vi "cube Controller.vi"(8 "error in":errorcluster) -> ()   [LabVIEW 2017]
doc: "This VI executes continuously carrying out the current operation and responding to updates or new operations. It will often contain the timing or control code that is difficult to place directly in TeleOp. This VI generally opens all sensors and motors and isolates the rest of the robot code from knowing how the operations are carried out."
uses:
  <vilib>/Rock Robotics/WPI/Framework/Completion Status.ctl
  cube Setpoints.ctl
  cube Operations.ctl
  <vilib>/Rock Robotics/SystemInterfaces/AI/FPGA_AIChannel.ctl
  Public/Documents/Cross The Road Electronics/Phoenix-LabVIEW/Motor Controller/Controls/CTRE_Phoenix_MotorControl_ControlMode.ctl
  cube Published Globals.vi
  Framework/Robot Global Data.vi
  <vilib>/Rock Robotics/Network Tables/NT Write Boolean.vi
panel:
  out "CubeLastCommandStatus":T1=enum."Incomplete"
  out "WaitTrigger":bool
  in  "Interactive Values":T2
  out "Current\nCmd":string
  in  "Buttons":cluster{"Execute Cmd":bool, "Abort Cmd":bool}
  out "Command Timing":cluster{"Start Time (ms)":u32, "Iterations":i32}
  out "Status":T1
  # "Tip: It may be helpful to observe inputs and sensor values.\nYou may also want to display tuning or debugging controls."
  # "Interactive Command: You may fill in the settings for a command\nand schedule it with the Execute button. You can observe and abort\nany command while fine tuning the code for the controller."
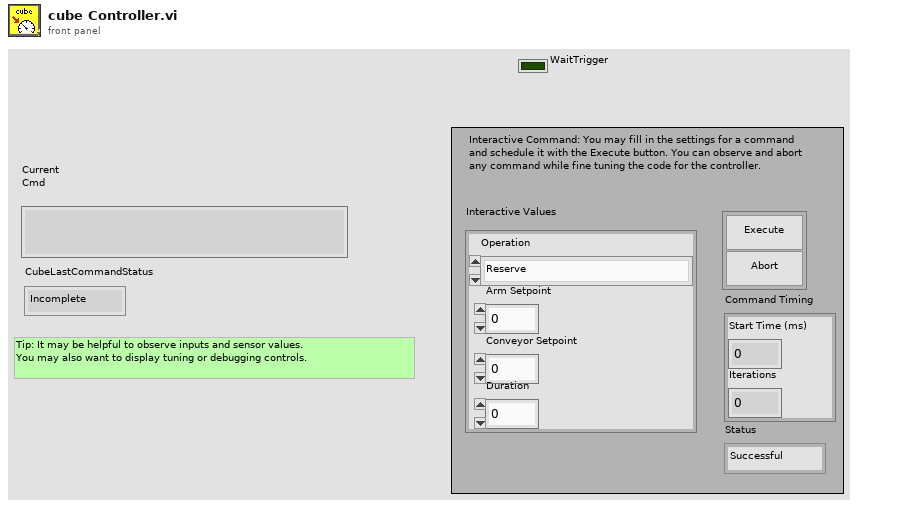
[diagram p1: front panel]
types:
  T1 = typedef "Completion Status.ctl" = enum16{"Successful", "Aborted", "Incomplete"}
  T2 = typedef "cube Setpoints.ctl" = cluster{"Operation":T3, "Arm Setpoint":dbl, "Duration":dbl, "Conveyor Setpoint":dbl}
  T3 = typedef "cube Operations.ctl" = enum16{"Reserve", "Read Current", "Immediate", "Chew", "Puke", "Swallow", "Poop", "SpitFast", "SpitSlow"}
  T4 = typedef "FPGA_AIChannel.ctl" = enum8{"AI 0", "AI 1", "AI 2", "AI 3", "AI MXP 0", "AI MXP 1", "AI MXP 2", "AI MXP 3", "Invalid"}
  T5 = typedef "WPI_AnalogChannelDevRef.ctl" = cluster{"DevStatus":errorcluster, "Analog Channel":T4}
  T6 = typedef "WPI_MotorControlDeviceRef.ctl" = cluster{"DeviceStatus":errorcluster, "Type":T7, "PWM":cluster{"PWM Channel":T8, "DeadBand":T9}, "CAN":cluster{"Device Number":u8, "SetOutput VI Ref":variant, "GetOutput VI Ref":variant, "Enable VI Ref":variant, "Disable VI Ref":variant, "Data":variant}, "Invert":bool, "DIO PWM":cluster{"PWM \"Enable\" Channel":T8, "DIOChannel":T10, "PWM Rate":dbl}}
  T7 = typedef "WPI_MotorControlType.ctl" = enum16{"PWM", "CAN", "DIO PWM"}
  T8 = typedef "FPGA_DIOPWMChannel.ctl" = enum8{"PWM 0", "PWM 1", "PWM 2", "PWM 3", "PWM 4", "PWM 5", "PWM 6", "PWM 7", "PWM 8", "PWM 9", "PWM MXP 0", "PWM MXP 1", "PWM MXP 2", "PWM MXP 3", "PWM MXP 4", "PWM MXP 5", "PWM MXP 6", "PWM MXP 7", "PWM MXP 8", "PWM MXP 9", "Invalid"}
  T9 = typedef "WPI_PWMDeadband.ctl" = cluster{"Name":string, "maxPositivePwm":i32, "minPositivePwm":i32, "centerPwm":i32, "maxNegativePwm":i32, "minNegativePwm":i32, "angularRange":u16}
  T10 = typedef "FPGA_DIOChannel.ctl" = enum8{"DIO 0", "DIO 1", "DIO 2", "DIO 3", "DIO 4", "DIO 5", "DIO 6", "DIO 7", "DIO 8", "DIO 9", "DIO MXP 0", "DIO MXP 1", "DIO MXP 2", "DIO MXP 3", "DIO MXP 4", "DIO MXP 5", "DIO MXP 6", "DIO MXP 7", "DIO MXP 8", "DIO MXP 9", "DIO MXP 10", "DIO MXP 11", "DIO MXP 12", "DIO MXP 13", "DIO MXP 14", "DIO MXP 15", "SPI Port CS1", "SPI Port CS2", "SPI Port CS3", "SPI Port MISO", "SPI Port MOSI", "Invalid"}
  T11 = typedef "FPGA_AnalogTriggerDevRef.ctl" = cluster{"DevStatus":errorcluster, "AnalogTriggerIndex":T12}
  T12 = typedef "FPGA_AnalogTriggerIndex.ctl" = enum8{"Trig 0", "Trig 1", "Trig 2", "Trig 3", "Trig 4", "Trig 5", "Trig 6", "Trig 7", "Invalid"}
  T13 = typedef "Command Status Info.ctl" = cluster{"Name":string, "Status":T1, "notifier out":T14}
  T14 = typedef "Completion Notifier.ctl" = refnum<notifier>
  T15 = cluster{"Current Command":T2, "Command Timing":cluster{"Start Time (ms)":u32, "Iterations":i32}, "Command Arguments":cluster{"Command Info":T13, "Description":string, "Default Command":T2, "queue out":refnum<queue>, "Subsystem Name":string}}
  T16 = typedef "CTRE_Phoenix_MotorControl_ControlMode.ctl" = u16
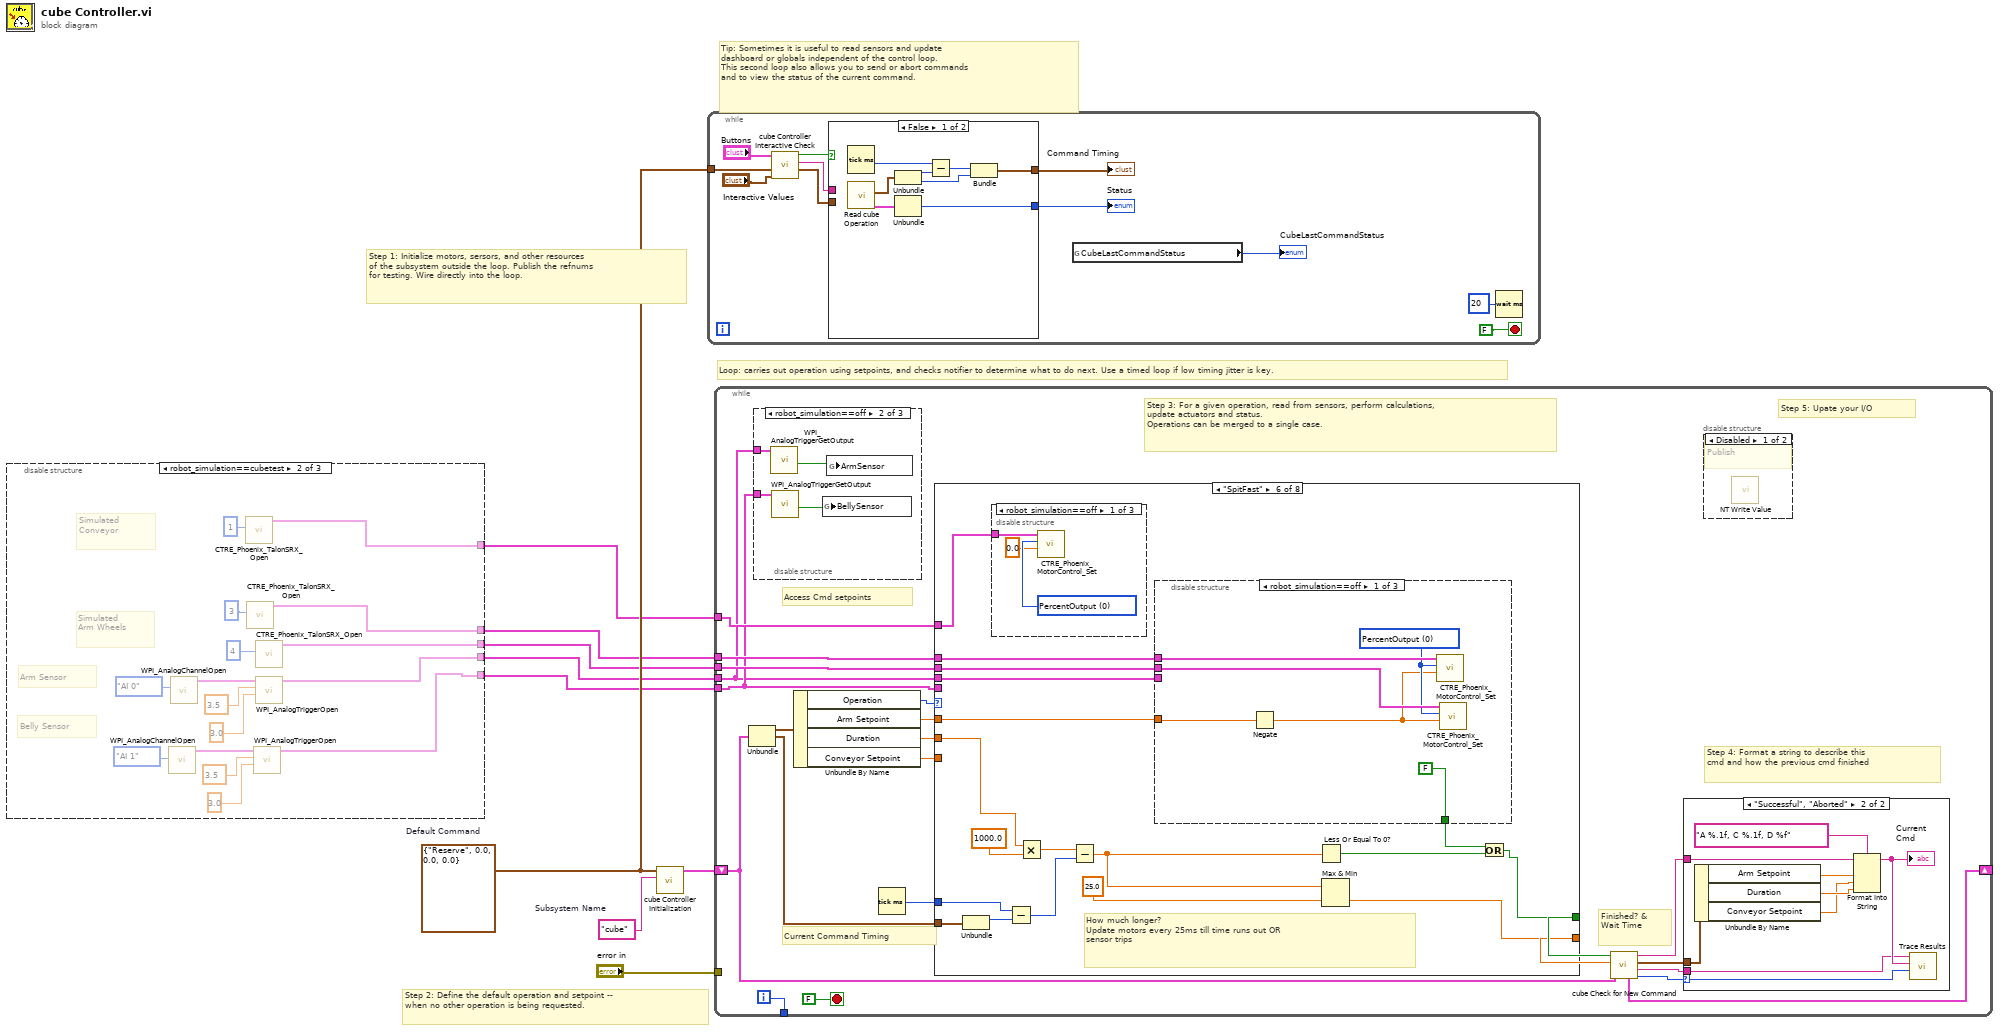
[diagram p0: block diagram]
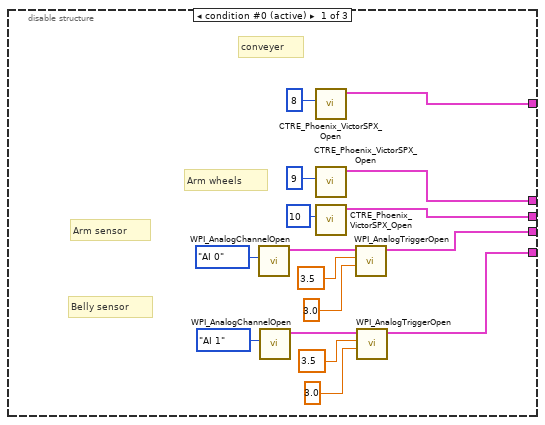
[diagram p2: hidden frame]
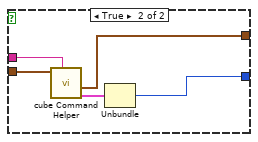
[diagram p4: hidden frame]
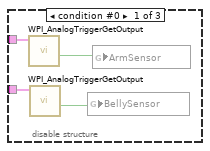
[diagram p5: hidden frame]
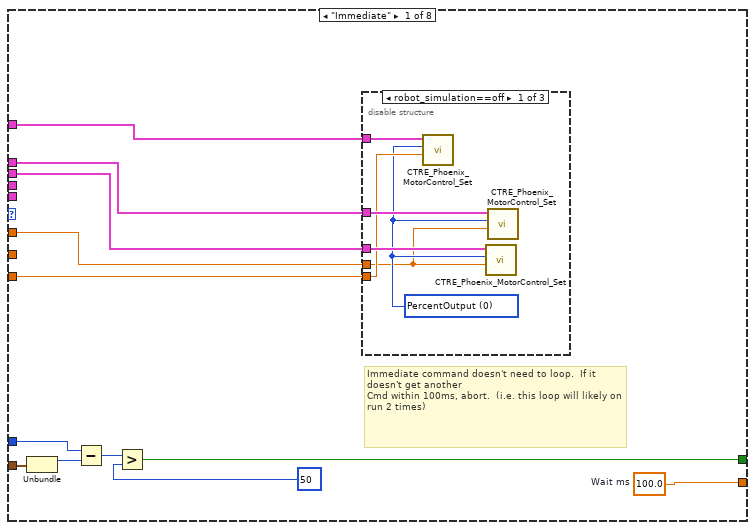
[diagram p9: hidden frame]
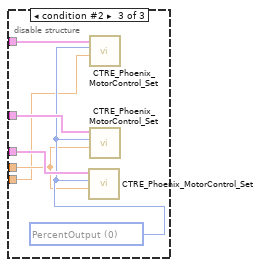
[diagram p11: hidden frame]
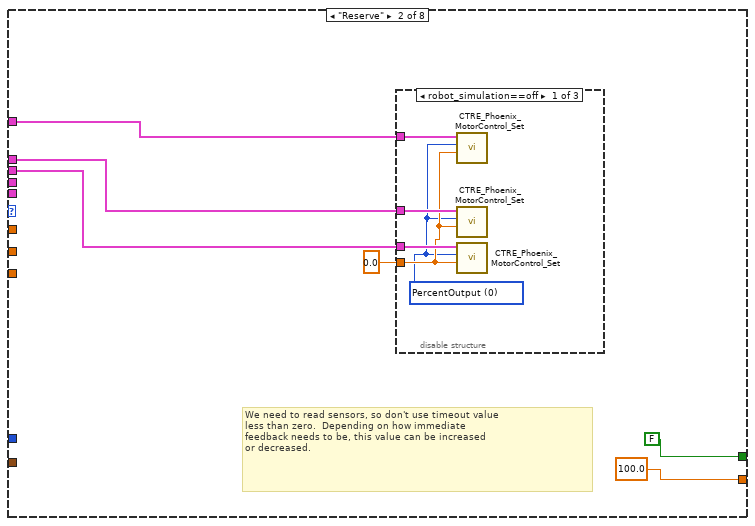
[diagram p12: hidden frame]
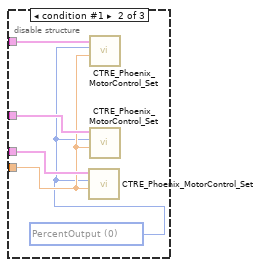
[diagram p13: hidden frame]
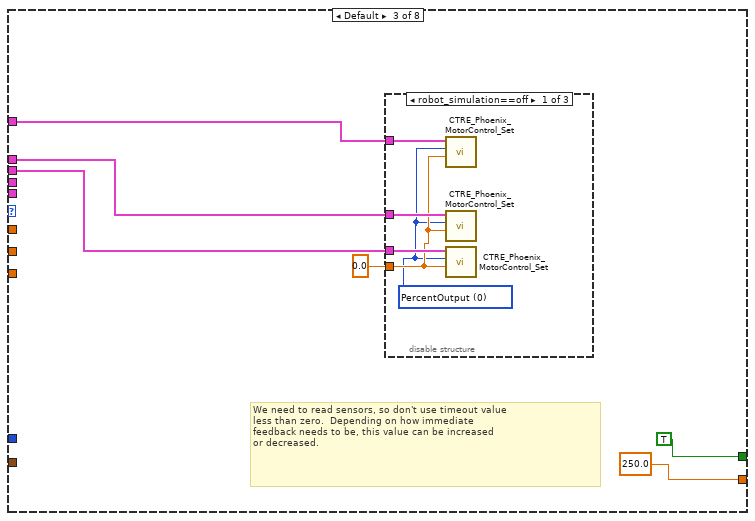
[diagram p15: hidden frame]
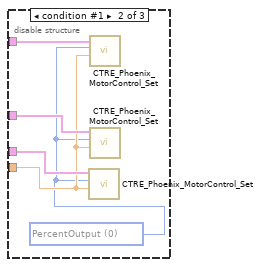
[diagram p16: hidden frame]
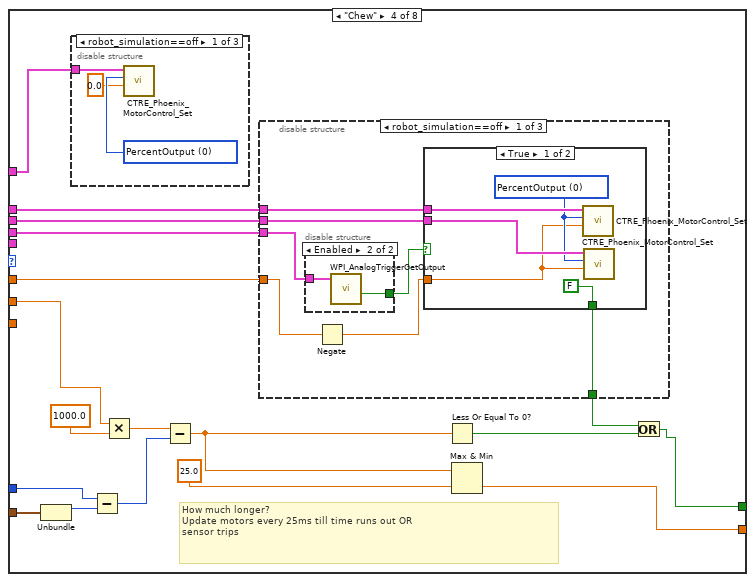
[diagram p18: hidden frame]
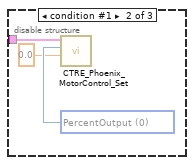
[diagram p19: hidden frame]
diagram:
  w6 = T2 {"Operation"=enum."Reserve", "Arm Setpoint"=0.0, "Duration"=0.0, "Conveyor Setpoint"=0.0}  # Default Command
  w7 = "cube"  # Subsystem Name
  # "Tip: Sometimes it is useful to read sensors and update\ndashboard or globals independent of the control loop.\nThis second loop also allows you to send or abort commands\nand to view the status of the current command."
  # "Step 2: Define the default operation and setpoint --\nwhen no other operation is being requested."
  # "Step 1: Initialize motors, sersors, and other resources\nof the subsystem outside the loop. Publish the refnums\nfor testing. Wire directly into the loop."
  # "Loop: carries out operation using setpoints, and checks notifier to determine what to do next. Use a timed loop if low timing jitter is key."
  n1 = disable-structure shown="robot_simulation==cubetest" {
    disable-tunnel: [w22 w38 _] -> w5
    disable-tunnel: [w21 w37 _] -> w4
    disable-tunnel: [w10 w36 _] -> w1
    disable-tunnel: [w16 w31 _] -> w3
    disable-tunnel: [w11 w26 _] -> w2
    frame condition #0 (active) {
      # "Belly sensor"
      # "Arm sensor"
      # "Arm wheels"
      # "conveyer"
      n2 = call <vilib>:"WPI_AnalogChannelOpen.vi"("Analog Channel"=FPGA_AIChannel."AI 0") -> ("AIDeviceRef"=w19:T5)  [unwired: 9 in, 1 out]
      n3 = call <vilib>:"WPI_AnalogChannelOpen.vi"("Analog Channel"=FPGA_AIChannel."AI 1") -> ("AIDeviceRef"=w14:T5)  [unwired: 9 in, 1 out]
      n4 = call "CTRE_Phoenix_VictorSPX_Open.vi"("Device Number"=u8 8) -> ("CAN Talon SRX Ref"=w10:T6)  [unwired: 9 in, 1 out]
      n5 = call "CTRE_Phoenix_VictorSPX_Open.vi"("Device Number"=u8 9) -> ("CAN Talon SRX Ref"=w22:T6)  [unwired: 9 in, 1 out]
      n6 = call "CTRE_Phoenix_VictorSPX_Open.vi"("Device Number"=u8 10) -> ("CAN Talon SRX Ref"=w21:T6)  [unwired: 9 in, 1 out]
      n7 = call <vilib>:"WPI_AnalogTriggerOpen.vi"("LowerLimit (v)"=3.0, "UpperLimit (v)"=3.5, "AnalogTriggerSource"=w19) -> ("AnalogTriggerDevRef"=w16:T11)  [unwired: 7 in, 1 out]
      n8 = call <vilib>:"WPI_AnalogTriggerOpen.vi"("LowerLimit (v)"=3.0, "UpperLimit (v)"=3.5, "AnalogTriggerSource"=w14) -> ("AnalogTriggerDevRef"=w11:T11)  [unwired: 7 in, 1 out]
    }
    frame condition #1 {
      # "Belly Sensor"
      # "Arm Sensor"
      # "Simulated\nConveyor"
      # "Simulated\nArm Wheels"
      n9 = call <vilib>:"WPI_AnalogChannelOpen.vi"("Analog Channel"=FPGA_AIChannel."AI 1") -> ("AIDeviceRef"=w29:T5)  [unwired: 9 in, 1 out]
      n10 = call <vilib>:"WPI_AnalogChannelOpen.vi"("Analog Channel"=FPGA_AIChannel."AI 0") -> ("AIDeviceRef"=w34:T5)  [unwired: 9 in, 1 out]
      n11 = call "CTRE_Phoenix_TalonSRX_Open.vi"("Device Number"=u8 1) -> ("CAN Talon SRX Ref"=w36:T6)  [unwired: 9 in, 1 out]
      n12 = call "CTRE_Phoenix_TalonSRX_Open.vi"("Device Number"=u8 3) -> ("CAN Talon SRX Ref"=w38:T6)  [unwired: 9 in, 1 out]
      n13 = call <vilib>:"WPI_AnalogTriggerOpen.vi"("LowerLimit (v)"=3.0, "UpperLimit (v)"=3.5, "AnalogTriggerSource"=w29) -> ("AnalogTriggerDevRef"=w26:T11)  [unwired: 7 in, 1 out]
      n14 = call "CTRE_Phoenix_TalonSRX_Open.vi"("Device Number"=u8 4) -> ("CAN Talon SRX Ref"=w37:T6)  [unwired: 9 in, 1 out]
      n15 = call <vilib>:"WPI_AnalogTriggerOpen.vi"("LowerLimit (v)"=3.0, "UpperLimit (v)"=3.5, "AnalogTriggerSource"=w34) -> ("AnalogTriggerDevRef"=w31:T11)  [unwired: 7 in, 1 out]
    }
    frame condition #2 {
    }
  }
  n16 = call "cube Controller Initialization.vi"("Subsystem Name"=w7, "Default Command"=w6) -> ("Current Command"=w8:T15)  [unwired: 9 in]
  n17 = while {
    tunnel: w6 -> [w49]
    stop <- FALSE stop-if-true
    n18 = call "cube Controller Interactive Check.vi"("Interactive Command in"="Interactive Values", "Default Command"=w49, "Buttons"="Buttons") -> ("Interactive Command out"=w46:T2, "Trace String"=w47:string, "Schedule"=w48:bool)  [unwired: 6 in]
    n19 = case shown="False" w48 {
      tunnel: [w60 w65] -> w45
      tunnel: w46 -> [_ w63]
      tunnel: [w56 w61] -> w44
      tunnel: w47 -> [_ w64]
      frame False {
        n20 = Tick Count (ms)() -> (millisecond timer value=w55:u32)
        n21 = call "Read cube Operation.vi"() -> ("Command Info"=w54:T13, "Command Timing"=w53:cluster{"Start Time (ms)":u32, "Iterations":i32})  [unwired: 9 in, 1 out]
        n22 = Unbundle(w53) -> ("Start Time (ms)"=w59:u32, "Iterations"=w57:i32)
        n23 = Unbundle(w54) -> ("Status"=w60:T1)  [unwired: 2 out]
        n24 = Subtract(x=w55, y=w59) -> (x-y=w58:u32)
        n25 = Bundle(w58, "Iterations"=w57) -> (w56:cluster{u32, "Iterations":i32})  [unwired: 1 in]
      }
      frame True {
        n26 = call "cube Command Helper.vi"("Description"=w64, "SubSystem Data"=w63) -> ("Command Info Out"=w62:T13, "Command Timing"=w61:cluster{"Start Time (ms)":u32, "Iterations":i32})  [unwired: 7 in, 1 out]
        n27 = Unbundle(w62) -> ("Status"=w65:T1)  [unwired: 2 out]
      }
    }
    "Status" <- w45
    "Command Timing" <- w44
    n28 = global read "cube Published Globals.vi" "CubeLastCommandStatus"() -> (→"CubeLastCommandStatus":T1)
    n29 = Wait (ms)(milliseconds to wait=u32 20) -> ()  [unwired: 1 out]
  }
  n30 = while {
    shift-right: [w83] -> _
    shift-left: w8 -> [w76]
    tunnel: [w86] -> _
    tunnel: "error in" -> [_]
    tunnel: w5 -> [w75]
    tunnel: w4 -> [w74]
    tunnel: w1 -> [w73]
    tunnel: w3 -> [w66]
    tunnel: w2 -> [w67]
    i -> [w86]
    stop <- FALSE stop-if-true
    # "Step 5: Upate your I/O"
    # "Step 4: Format a string to describe this\ncmd and how the previous cmd finished"
    # "Current Command Timing"
    # "Access Cmd setpoints"
    # "Finished? &\nWait Time"
    # "Step 3: For a given operation, read from sensors, perform calculations,\nupdate actuators and status.\nOperations can be merged to a single case."
    n31 = Unbundle(w76) -> ("Current Command"=w72:T2, "Command Timing"=w84:cluster{"Start Time (ms)":u32, "Iterations":i32})  [unwired: 1 out]
    n32 = disable-structure shown="robot_simulation==off" {
      disable-tunnel: w67 -> [w88 w93 _]
      disable-tunnel: w66 -> [w89 w92 _]
      frame condition #0 {
        n33 = call <vilib>:"WPI_AnalogTriggerGetOutput.vi"("AnalogTriggerDevRef"=w89) -> ("Trigger State"=w91:bool)  [unwired: 7 in, 3 out]
        n34 = call <vilib>:"WPI_AnalogTriggerGetOutput.vi"("AnalogTriggerDevRef"=w88) -> ("Trigger State"=w90:bool)  [unwired: 7 in, 3 out]
        n35 = global write "Robot Global Data.vi" "BellySensor"(w90) -> ()
        n36 = global write "Robot Global Data.vi" "ArmSensor"(w91) -> ()
      }
      frame condition #1 (active) {
        n37 = call <vilib>:"WPI_AnalogTriggerGetOutput.vi"("AnalogTriggerDevRef"=w92) -> ("Trigger State"=w95:bool)  [unwired: 7 in, 3 out]
        n38 = call <vilib>:"WPI_AnalogTriggerGetOutput.vi"("AnalogTriggerDevRef"=w93) -> ("Trigger State"=w94:bool)  [unwired: 7 in, 3 out]
        n39 = global write "Robot Global Data.vi" "BellySensor"(w94) -> ()
        n40 = global write "Robot Global Data.vi" "ArmSensor"(w95) -> ()
      }
      frame condition #2 {
      }
    }
    n41 = Unbundle By Name(w72) -> ("Operation"=w71:T3, "Arm Setpoint"=w70:dbl, "Duration"=w69:dbl, "Conveyor Setpoint"=w68:dbl)
    n42 = Tick Count (ms)() -> (millisecond timer value=w85:u32)
    n43 = case shown="\"SpitFast\"" w71 {
      tunnel: [w116 100.0 250.0 ("Infinite") w170 w231 w267 w304 w372] -> w81
      tunnel: [w110 FALSE ("ignore previous (F)") TRUE ("ignore previous (F)") w165 w227 w262 w300 w368] -> w82
      tunnel: w84 -> [w112 _ _ w172 w233 w269 w306 w374]
      tunnel: w85 -> [w111 _ _ w171 w232 w268 w305 w373]
      tunnel: w75 -> [w108 w131 w147 w169 w230 w266 w303 w371]
      tunnel: w74 -> [w107 w130 w146 w168 w229 w265 w302 w370]
      tunnel: w73 -> [w109 w132 w148 w161 w222 w258 w295 w364]
      tunnel: w70 -> [w106 _ _ w162 w224 w259 w297 w365]
      tunnel: w69 -> [_ _ _ w167 w228 w264 w301 w369]
      tunnel: w68 -> [w105 _ _ _ w221 _ w294 w363]
      tunnel: w66 -> [_ _ _ w166 _ w263 _ w358]
      tunnel: w67 -> [_ _ _ _ w223 _ w296 w362]
      frame "Immediate" {
        w116 = 100.0  # Wait ms
        # "Immediate command doesn't need to loop.  If it doesn't get another\nCmd within 100ms, abort.  (i.e. this loop will likely on run 2 times)"
        n44 = Unbundle(w112) -> ("Start Time (ms)"=w115:u32)  [unwired: 1 out]
        n45 = Subtract(x=w111, y=w115) -> (x-y=w114:u32)
        n46 = Greater?(x=w114, y=u8 50 ("Left Motor")) -> (0:w110:bool)
        n47 = disable-structure shown="robot_simulation==off" {
          disable-tunnel: w109 -> [w122 _ w128]
          disable-tunnel: w108 -> [w121 _ w127]
          disable-tunnel: w107 -> [w120 _ w126]
          disable-tunnel: w106 -> [w117 _ w124]
          disable-tunnel: w105 -> [w119 _ w123]
          frame condition #0 (active) {
            w118 = T16 0 items=["PercentOutput"=0, "Position"=1, "Velocity"=2, "Current"=3, "Follower"=5, "MotionProfile"=6, "MotionMagic"=7, "MotionMagicArc"=8, "MotionProfileArc"=10, "Disabled"=15] ("Control Mode")
            n48 = call "CTRE_Phoenix_MotorControl_Set.vi"("Output"=w119, "Control Mode"=w118, "PhoenixMotorControlDevRef"=w122) -> ()  [unwired: 7 in, 2 out]
            n49 = call "CTRE_Phoenix_MotorControl_Set.vi"("Output"=w117, "Control Mode"=w118, "PhoenixMotorControlDevRef"=w120) -> ()  [unwired: 7 in, 2 out]
            n50 = call "CTRE_Phoenix_MotorControl_Set.vi"("Output"=w117, "Control Mode"=w118, "PhoenixMotorControlDevRef"=w121) -> ()  [unwired: 7 in, 2 out]
          }
          frame condition #1 {
          }
          frame condition #2 {
            w125 = T16 0 items=["PercentOutput"=0, "Position"=1, "Velocity"=2, "Current"=3, "Follower"=5, "MotionProfile"=6, "MotionMagic"=7, "MotionMagicArc"=8, "MotionProfileArc"=10, "Disabled"=15] ("Control Mode")
            n51 = call "CTRE_Phoenix_MotorControl_Set.vi"("Output"=w124, "Control Mode"=w125, "PhoenixMotorControlDevRef"=w126) -> ()  [unwired: 7 in, 2 out]
            n52 = call "CTRE_Phoenix_MotorControl_Set.vi"("Output"=w123, "Control Mode"=w125, "PhoenixMotorControlDevRef"=w128) -> ()  [unwired: 7 in, 2 out]
            n53 = call "CTRE_Phoenix_MotorControl_Set.vi"("Output"=w124, "Control Mode"=w125, "PhoenixMotorControlDevRef"=w127) -> ()  [unwired: 7 in, 2 out]
          }
        }
      }
      frame "Reserve" {
        # "We need to read sensors, so don't use timeout value\nless than zero.  Depending on how immediate \nfeedback needs to be, this value can be increased\nor decreased."
        n54 = disable-structure shown="robot_simulation==off" {
          disable-tunnel: w132 -> [w139 w144 _]
          disable-tunnel: w131 -> [w138 w143 _]
          disable-tunnel: w130 -> [w137 w142 _]
          disable-tunnel: 0.0 ("Setpoint") -> [w136 w141 _]
          frame condition #0 (active) {
            w135 = T16 0 items=["PercentOutput"=0, "Position"=1, "Velocity"=2, "Current"=3, "Follower"=5, "MotionProfile"=6, "MotionMagic"=7, "MotionMagicArc"=8, "MotionProfileArc"=10, "Disabled"=15] ("Control Mode")
            n55 = call "CTRE_Phoenix_MotorControl_Set.vi"("Output"=w136, "Control Mode"=w135, "PhoenixMotorControlDevRef"=w139) -> ()  [unwired: 7 in, 2 out]
            n56 = call "CTRE_Phoenix_MotorControl_Set.vi"("Output"=w136, "Control Mode"=w135, "PhoenixMotorControlDevRef"=w138) -> ()  [unwired: 7 in, 2 out]
            n57 = call "CTRE_Phoenix_MotorControl_Set.vi"("Output"=w136, "Control Mode"=w135, "PhoenixMotorControlDevRef"=w137) -> ()  [unwired: 7 in, 2 out]
          }
          frame condition #1 {
            w140 = T16 0 items=["PercentOutput"=0, "Position"=1, "Velocity"=2, "Current"=3, "Follower"=5, "MotionProfile"=6, "MotionMagic"=7, "MotionMagicArc"=8, "MotionProfileArc"=10, "Disabled"=15] ("Control Mode")
            n58 = call "CTRE_Phoenix_MotorControl_Set.vi"("Output"=w141, "Control Mode"=w140, "PhoenixMotorControlDevRef"=w142) -> ()  [unwired: 7 in, 2 out]
            n59 = call "CTRE_Phoenix_MotorControl_Set.vi"("Output"=w141, "Control Mode"=w140, "PhoenixMotorControlDevRef"=w144) -> ()  [unwired: 7 in, 2 out]
            n60 = call "CTRE_Phoenix_MotorControl_Set.vi"("Output"=w141, "Control Mode"=w140, "PhoenixMotorControlDevRef"=w143) -> ()  [unwired: 7 in, 2 out]
          }
          frame condition #2 {
          }
        }
      }
      frame Default {
        # "We need to read sensors, so don't use timeout value\nless than zero.  Depending on how immediate \nfeedback needs to be, this value can be increased\nor decreased."
        n61 = disable-structure shown="robot_simulation==off" {
          disable-tunnel: w148 -> [w155 w160 _]
          disable-tunnel: w147 -> [w154 w159 _]
          disable-tunnel: w146 -> [w153 w158 _]
          disable-tunnel: 0.0 ("Setpoint") -> [w152 w157 _]
          frame condition #0 (active) {
            w151 = T16 0 items=["PercentOutput"=0, "Position"=1, "Velocity"=2, "Current"=3, "Follower"=5, "MotionProfile"=6, "MotionMagic"=7, "MotionMagicArc"=8, "MotionProfileArc"=10, "Disabled"=15] ("Control Mode")
            n62 = call "CTRE_Phoenix_MotorControl_Set.vi"("Output"=w152, "Control Mode"=w151, "PhoenixMotorControlDevRef"=w155) -> ()  [unwired: 7 in, 2 out]
            n63 = call "CTRE_Phoenix_MotorControl_Set.vi"("Output"=w152, "Control Mode"=w151, "PhoenixMotorControlDevRef"=w154) -> ()  [unwired: 7 in, 2 out]
            n64 = call "CTRE_Phoenix_MotorControl_Set.vi"("Output"=w152, "Control Mode"=w151, "PhoenixMotorControlDevRef"=w153) -> ()  [unwired: 7 in, 2 out]
          }
          frame condition #1 {
            w156 = T16 0 items=["PercentOutput"=0, "Position"=1, "Velocity"=2, "Current"=3, "Follower"=5, "MotionProfile"=6, "MotionMagic"=7, "MotionMagicArc"=8, "MotionProfileArc"=10, "Disabled"=15] ("Control Mode")
            n65 = call "CTRE_Phoenix_MotorControl_Set.vi"("Output"=w157, "Control Mode"=w156, "PhoenixMotorControlDevRef"=w158) -> ()  [unwired: 7 in, 2 out]
            n66 = call "CTRE_Phoenix_MotorControl_Set.vi"("Output"=w157, "Control Mode"=w156, "PhoenixMotorControlDevRef"=w160) -> ()  [unwired: 7 in, 2 out]
            n67 = call "CTRE_Phoenix_MotorControl_Set.vi"("Output"=w157, "Control Mode"=w156, "PhoenixMotorControlDevRef"=w159) -> ()  [unwired: 7 in, 2 out]
          }
          frame condition #2 {
          }
        }
      }
      frame "Chew" {
        # "How much longer?\nUpdate motors every 25ms till time runs out OR\nsensor trips"
        n68 = Unbundle(w172) -> ("Start Time (ms)"=w175:u32)  [unwired: 1 out]
        n69 = disable-structure shown="robot_simulation==off" {
          disable-tunnel: w161 -> [w180 w183 _]
          frame condition #0 (active) {
            w181 = T16 0 items=["PercentOutput"=0, "Position"=1, "Velocity"=2, "Current"=3, "Follower"=5, "MotionProfile"=6, "MotionMagic"=7, "MotionMagicArc"=8, "MotionProfileArc"=10, "Disabled"=15] ("Control Mode")
            n70 = call "CTRE_Phoenix_MotorControl_Set.vi"("Output"=0.0, "Control Mode"=w181, "PhoenixMotorControlDevRef"=w180) -> ()  [unwired: 7 in, 2 out]
          }
          frame condition #1 {
            w184 = T16 0 items=["PercentOutput"=0, "Position"=1, "Velocity"=2, "Current"=3, "Follower"=5, "MotionProfile"=6, "MotionMagic"=7, "MotionMagicArc"=8, "MotionProfileArc"=10, "Disabled"=15] ("Control Mode")
            n71 = call "CTRE_Phoenix_MotorControl_Set.vi"("Output"=0.0, "Control Mode"=w184, "PhoenixMotorControlDevRef"=w183) -> ()  [unwired: 7 in, 2 out]
          }
          frame condition #2 {
          }
        }
        n72 = Subtract(x=w171, y=w175) -> (x-y=w178:u32)
        n73 = Multiply(x=w167, y=1000.0) -> (x*y=w177:dbl)
        n74 = Subtract(x=w177, y=w178) -> (x-y=w174:dbl)
        n75 = disable-structure shown="robot_simulation==off" {
          disable-tunnel: w169 -> [w191 w210 _]
          disable-tunnel: w168 -> [w190 w209 _]
          disable-tunnel: w162 -> [w185 w208 _]
          disable-tunnel: w166 -> [w189 w207 _]
          disable-tunnel: [w187 w205 _] -> w163
          frame condition #0 (active) {
            n76 = disable-structure shown="Enabled" {
              disable-tunnel: w189 -> [_ w194]
              disable-tunnel: [TRUE ("Trigger State") w193] -> w188
              frame Disabled {
              }
              frame Enabled {
                n77 = call <vilib>:"WPI_AnalogTriggerGetOutput.vi"("AnalogTriggerDevRef"=w194) -> ("Trigger State"=w193:bool)  [unwired: 7 in, 3 out]
              }
            }
            n78 = Negate(x=w185) -> (-x=w186:dbl)
            n79 = case shown="True" w188 {
              tunnel: w191 -> [w199 w204]
              tunnel: w190 -> [w198 w203]
              tunnel: w186 -> [w195 _]
              tunnel: [FALSE TRUE] -> w187
              frame True {
                w197 = T16 0 items=["PercentOutput"=0, "Position"=1, "Velocity"=2, "Current"=3, "Follower"=5, "MotionProfile"=6, "MotionMagic"=7, "MotionMagicArc"=8, "MotionProfileArc"=10, "Disabled"=15] ("Control Mode")
                n80 = call "CTRE_Phoenix_MotorControl_Set.vi"("Output"=w195, "Control Mode"=w197, "PhoenixMotorControlDevRef"=w199) -> ()  [unwired: 7 in, 2 out]
                n81 = call "CTRE_Phoenix_MotorControl_Set.vi"("Output"=w195, "Control Mode"=w197, "PhoenixMotorControlDevRef"=w198) -> ()  [unwired: 7 in, 2 out]
              }
              frame False {
                w201 = 0.0 ("Output")
                w202 = T16 0 items=["PercentOutput"=0, "Position"=1, "Velocity"=2, "Current"=3, "Follower"=5, "MotionProfile"=6, "MotionMagic"=7, "MotionMagicArc"=8, "MotionProfileArc"=10, "Disabled"=15] ("Control Mode")
                n82 = call "CTRE_Phoenix_MotorControl_Set.vi"("Output"=w201, "Control Mode"=w202, "PhoenixMotorControlDevRef"=w204) -> ()  [unwired: 7 in, 2 out]
                n83 = call "CTRE_Phoenix_MotorControl_Set.vi"("Output"=w201, "Control Mode"=w202, "PhoenixMotorControlDevRef"=w203) -> ()  [unwired: 7 in, 2 out]
              }
            }
          }
          frame condition #1 {
            n84 = call <vilib>:"WPI_AnalogTriggerGetOutput.vi"("AnalogTriggerDevRef"=w207) -> ("Trigger State"=w206:bool)  [unwired: 7 in, 3 out]
            n85 = case shown="True" w206 {
              tunnel: w210 -> [w214 w220]
              tunnel: w209 -> [w213 w219]
              tunnel: w208 -> [w211 _]
              tunnel: [FALSE TRUE] -> w205
              frame True {
                w212 = T16 0 items=["PercentOutput"=0, "Position"=1, "Velocity"=2, "Current"=3, "Follower"=5, "MotionProfile"=6, "MotionMagic"=7, "MotionMagicArc"=8, "MotionProfileArc"=10, "Disabled"=15] ("Control Mode")
                n86 = call "CTRE_Phoenix_MotorControl_Set.vi"("Output"=w211, "Control Mode"=w212, "PhoenixMotorControlDevRef"=w214) -> ()  [unwired: 7 in, 2 out]
                n87 = call "CTRE_Phoenix_MotorControl_Set.vi"("Output"=w211, "Control Mode"=w212, "PhoenixMotorControlDevRef"=w213) -> ()  [unwired: 7 in, 2 out]
              }
              frame False {
                w218 = T16 0 items=["PercentOutput"=0, "Position"=1, "Velocity"=2, "Current"=3, "Follower"=5, "MotionProfile"=6, "MotionMagic"=7, "MotionMagicArc"=8, "MotionProfileArc"=10, "Disabled"=15] ("Control Mode")
                w217 = 0.0 ("Output")
                n88 = call "CTRE_Phoenix_MotorControl_Set.vi"("Output"=w217, "Control Mode"=w218, "PhoenixMotorControlDevRef"=w220) -> ()  [unwired: 7 in, 2 out]
                n89 = call "CTRE_Phoenix_MotorControl_Set.vi"("Output"=w217, "Control Mode"=w218, "PhoenixMotorControlDevRef"=w219) -> ()  [unwired: 7 in, 2 out]
              }
            }
          }
          frame condition #2 {
          }
        }
        n90 = Less Or Equal To 0?(x=w174) -> (x <= 0?=w164:bool)
        n91 = Max & Min(x=w174, y=25.0) -> (min(x,y)=w170:dbl)  [unwired: 1 out]
        n92 = Or(x=w163, y=w164) -> (x .or. y?=w165:bool)
      }
      frame "Poop" {
        # "How much longer?\nUpdate motors every 25ms till time runs out OR\nsensor trips"
        n93 = Unbundle(w233) -> ("Start Time (ms)"=w236:u32)  [unwired: 1 out]
        n94 = Subtract(x=w232, y=w236) -> (x-y=w239:u32)
        n95 = Multiply(x=w228, y=1000.0) -> (x*y=w238:dbl)
        n96 = Subtract(x=w238, y=w239) -> (x-y=w235:dbl)
        n97 = disable-structure shown="robot_simulation==off" {
          disable-tunnel: w230 -> [w247 w257 _]
          disable-tunnel: w229 -> [w246 w256 _]
          disable-tunnel: w224 -> [w244 w252 _]
          disable-tunnel: w223 -> [_ _ _]
          disable-tunnel: [FALSE FALSE _] -> w225
          disable-tunnel: w222 -> [w248 w254 _]
          disable-tunnel: w221 -> [w243 w251 _]
          frame condition #0 (active) {
            w241 = T16 0 items=["PercentOutput"=0, "Position"=1, "Velocity"=2, "Current"=3, "Follower"=5, "MotionProfile"=6, "MotionMagic"=7, "MotionMagicArc"=8, "MotionProfileArc"=10, "Disabled"=15] ("Control Mode")
            n98 = Negate(x=w244) -> (-x=w240:dbl)
            n99 = Negate(x=w243) -> (-x=w242:dbl)
            n100 = call "CTRE_Phoenix_MotorControl_Set.vi"("Output"=w240, "Control Mode"=w241, "PhoenixMotorControlDevRef"=w247) -> ()  [unwired: 7 in, 2 out]
            n101 = call "CTRE_Phoenix_MotorControl_Set.vi"("Output"=w240, "Control Mode"=w241, "PhoenixMotorControlDevRef"=w246) -> ()  [unwired: 7 in, 2 out]
            n102 = call "CTRE_Phoenix_MotorControl_Set.vi"("Output"=w242, "Control Mode"=w241, "PhoenixMotorControlDevRef"=w248) -> ()  [unwired: 7 in, 2 out]
          }
          frame condition #1 {
            w253 = T16 0 items=["PercentOutput"=0, "Position"=1, "Velocity"=2, "Current"=3, "Follower"=5, "MotionProfile"=6, "MotionMagic"=7, "MotionMagicArc"=8, "MotionProfileArc"=10, "Disabled"=15] ("Control Mode")
            n103 = Negate(x=w252) -> (-x=w249:dbl)
            n104 = Negate(x=w251) -> (-x=w250:dbl)
            n105 = call "CTRE_Phoenix_MotorControl_Set.vi"("Output"=w249, "Control Mode"=w253, "PhoenixMotorControlDevRef"=w257) -> ()  [unwired: 7 in, 2 out]
            n106 = call "CTRE_Phoenix_MotorControl_Set.vi"("Output"=w249, "Control Mode"=w253, "PhoenixMotorControlDevRef"=w256) -> ()  [unwired: 7 in, 2 out]
            n107 = call "CTRE_Phoenix_MotorControl_Set.vi"("Output"=w250, "Control Mode"=w253, "PhoenixMotorControlDevRef"=w254) -> ()  [unwired: 7 in, 2 out]
          }
          frame condition #2 {
          }
        }
        n108 = Less Or Equal To 0?(x=w235) -> (x <= 0?=w226:bool)
        n109 = Max & Min(x=w235, y=25.0) -> (min(x,y)=w231:dbl)  [unwired: 1 out]
        n110 = Or(x=w225, y=w226) -> (x .or. y?=w227:bool)
      }
      frame "SpitFast" {
        # "How much longer?\nUpdate motors every 25ms till time runs out OR\nsensor trips"
        n111 = Unbundle(w269) -> ("Start Time (ms)"=w272:u32)  [unwired: 1 out]
        n112 = disable-structure shown="robot_simulation==off" {
          disable-tunnel: w258 -> [w277 w280 _]
          frame condition #0 (active) {
            w278 = T16 0 items=["PercentOutput"=0, "Position"=1, "Velocity"=2, "Current"=3, "Follower"=5, "MotionProfile"=6, "MotionMagic"=7, "MotionMagicArc"=8, "MotionProfileArc"=10, "Disabled"=15] ("Control Mode")
            n113 = call "CTRE_Phoenix_MotorControl_Set.vi"("Output"=0.0, "Control Mode"=w278, "PhoenixMotorControlDevRef"=w277) -> ()  [unwired: 7 in, 2 out]
          }
          frame condition #1 {
            w281 = T16 0 items=["PercentOutput"=0, "Position"=1, "Velocity"=2, "Current"=3, "Follower"=5, "MotionProfile"=6, "MotionMagic"=7, "MotionMagicArc"=8, "MotionProfileArc"=10, "Disabled"=15] ("Control Mode")
            n114 = call "CTRE_Phoenix_MotorControl_Set.vi"("Output"=0.0, "Control Mode"=w281, "PhoenixMotorControlDevRef"=w280) -> ()  [unwired: 7 in, 2 out]
          }
          frame condition #2 {
          }
        }
        n115 = Subtract(x=w268, y=w272) -> (x-y=w275:u32)
        n116 = Multiply(x=w264, y=1000.0) -> (x*y=w274:dbl)
        n117 = Subtract(x=w274, y=w275) -> (x-y=w271:dbl)
        n118 = disable-structure shown="robot_simulation==off" {
          disable-tunnel: w266 -> [w287 w293 _]
          disable-tunnel: w265 -> [w286 w292 _]
          disable-tunnel: w259 -> [w282 w290 _]
          disable-tunnel: w263 -> [_ _ _]
          disable-tunnel: [FALSE FALSE _] -> w260
          frame condition #0 (active) {
            w284 = T16 0 items=["PercentOutput"=0, "Position"=1, "Velocity"=2, "Current"=3, "Follower"=5, "MotionProfile"=6, "MotionMagic"=7, "MotionMagicArc"=8, "MotionProfileArc"=10, "Disabled"=15] ("Control Mode")
            n119 = Negate(x=w282) -> (-x=w283:dbl)
            n120 = call "CTRE_Phoenix_MotorControl_Set.vi"("Output"=w283, "Control Mode"=w284, "PhoenixMotorControlDevRef"=w287) -> ()  [unwired: 7 in, 2 out]
            n121 = call "CTRE_Phoenix_MotorControl_Set.vi"("Output"=w283, "Control Mode"=w284, "PhoenixMotorControlDevRef"=w286) -> ()  [unwired: 7 in, 2 out]
          }
          frame condition #1 {
            w289 = T16 0 items=["PercentOutput"=0, "Position"=1, "Velocity"=2, "Current"=3, "Follower"=5, "MotionProfile"=6, "MotionMagic"=7, "MotionMagicArc"=8, "MotionProfileArc"=10, "Disabled"=15] ("Control Mode")
            n122 = Negate(x=w290) -> (-x=w288:dbl)
            n123 = call "CTRE_Phoenix_MotorControl_Set.vi"("Output"=w288, "Control Mode"=w289, "PhoenixMotorControlDevRef"=w293) -> ()  [unwired: 7 in, 2 out]
            n124 = call "CTRE_Phoenix_MotorControl_Set.vi"("Output"=w288, "Control Mode"=w289, "PhoenixMotorControlDevRef"=w292) -> ()  [unwired: 7 in, 2 out]
          }
          frame condition #2 {
          }
        }
        n125 = Less Or Equal To 0?(x=w271) -> (x <= 0?=w261:bool)
        n126 = Max & Min(x=w271, y=25.0) -> (min(x,y)=w267:dbl)  [unwired: 1 out]
        n127 = Or(x=w260, y=w261) -> (x .or. y?=w262:bool)
      }
      frame "Swallow" {
        # "How much longer?\nUpdate motors every 25ms till time runs out OR\nsensor trips"
        n128 = Unbundle(w306) -> ("Start Time (ms)"=w309:u32)  [unwired: 1 out]
        n129 = Subtract(x=w305, y=w309) -> (x-y=w312:u32)
        n130 = Multiply(x=w301, y=1000.0) -> (x*y=w311:dbl)
        n131 = Subtract(x=w311, y=w312) -> (x-y=w308:dbl)
        n132 = disable-structure shown="robot_simulation==off" {
          disable-tunnel: w303 -> [w320 w343 _]
          disable-tunnel: w302 -> [w319 w342 _]
          disable-tunnel: w297 -> [w316 w341 _]
          disable-tunnel: w296 -> [w322 w340 _]
          disable-tunnel: [w318 w338 _] -> w298
          disable-tunnel: w295 -> [w321 w337 _]
          disable-tunnel: w294 -> [w314 w336 _]
          frame condition #0 (active) {
            n133 = Negate(x=w316) -> (-x=w315:dbl)
            n134 = Negate(x=w314) -> (-x=w313:dbl)
            n135 = call <vilib>:"WPI_AnalogTriggerGetOutput.vi"("AnalogTriggerDevRef"=w322) -> ("Trigger State"=w317:bool)  [unwired: 7 in, 3 out]
            n136 = case shown="True" w317 {
              tunnel: w320 -> [w328 w335]
              tunnel: w319 -> [w327 w334]
              tunnel: w315 -> [w323 _]
              tunnel: [FALSE TRUE] -> w318
              tunnel: w321 -> [w326 w332]
              tunnel: w313 -> [w324 _]
              frame True {
                w325 = T16 0 items=["PercentOutput"=0, "Position"=1, "Velocity"=2, "Current"=3, "Follower"=5, "MotionProfile"=6, "MotionMagic"=7, "MotionMagicArc"=8, "MotionProfileArc"=10, "Disabled"=15] ("Control Mode")
                n137 = call "CTRE_Phoenix_MotorControl_Set.vi"("Output"=w323, "Control Mode"=w325, "PhoenixMotorControlDevRef"=w328) -> ()  [unwired: 7 in, 2 out]
                n138 = call "CTRE_Phoenix_MotorControl_Set.vi"("Output"=w323, "Control Mode"=w325, "PhoenixMotorControlDevRef"=w327) -> ()  [unwired: 7 in, 2 out]
                n139 = call "CTRE_Phoenix_MotorControl_Set.vi"("Output"=w324, "Control Mode"=w325, "PhoenixMotorControlDevRef"=w326) -> ()  [unwired: 7 in, 2 out]
              }
              frame False {
                w330 = T16 0 items=["PercentOutput"=0, "Position"=1, "Velocity"=2, "Current"=3, "Follower"=5, "MotionProfile"=6, "MotionMagic"=7, "MotionMagicArc"=8, "MotionProfileArc"=10, "Disabled"=15] ("Control Mode")
                w331 = 0.0 ("Output")
                n140 = call "CTRE_Phoenix_MotorControl_Set.vi"("Output"=w331, "Control Mode"=w330, "PhoenixMotorControlDevRef"=w332) -> ()  [unwired: 7 in, 2 out]
                n141 = call "CTRE_Phoenix_MotorControl_Set.vi"("Output"=w331, "Control Mode"=w330, "PhoenixMotorControlDevRef"=w335) -> ()  [unwired: 7 in, 2 out]
                n142 = call "CTRE_Phoenix_MotorControl_Set.vi"("Output"=w331, "Control Mode"=w330, "PhoenixMotorControlDevRef"=w334) -> ()  [unwired: 7 in, 2 out]
              }
            }
          }
          frame condition #1 {
            n143 = call <vilib>:"WPI_AnalogTriggerGetOutput.vi"("AnalogTriggerDevRef"=w340) -> ("Trigger State"=w339:bool)  [unwired: 7 in, 3 out]
            n144 = case shown="True" w339 {
              tunnel: w343 -> [w349 w356]
              tunnel: w342 -> [w348 w355]
              tunnel: w341 -> [w344 _]
              tunnel: [FALSE TRUE] -> w338
              tunnel: w337 -> [w347 w353]
              tunnel: w336 -> [w345 _]
              frame True {
                w346 = T16 0 items=["PercentOutput"=0, "Position"=1, "Velocity"=2, "Current"=3, "Follower"=5, "MotionProfile"=6, "MotionMagic"=7, "MotionMagicArc"=8, "MotionProfileArc"=10, "Disabled"=15] ("Control Mode")
                n145 = call "CTRE_Phoenix_MotorControl_Set.vi"("Output"=w344, "Control Mode"=w346, "PhoenixMotorControlDevRef"=w349) -> ()  [unwired: 7 in, 2 out]
                n146 = call "CTRE_Phoenix_MotorControl_Set.vi"("Output"=w344, "Control Mode"=w346, "PhoenixMotorControlDevRef"=w348) -> ()  [unwired: 7 in, 2 out]
                n147 = call "CTRE_Phoenix_MotorControl_Set.vi"("Output"=w345, "Control Mode"=w346, "PhoenixMotorControlDevRef"=w347) -> ()  [unwired: 7 in, 2 out]
              }
              frame False {
                w351 = T16 0 items=["PercentOutput"=0, "Position"=1, "Velocity"=2, "Current"=3, "Follower"=5, "MotionProfile"=6, "MotionMagic"=7, "MotionMagicArc"=8, "MotionProfileArc"=10, "Disabled"=15] ("Control Mode")
                w352 = 0.0 ("Output")
                n148 = call "CTRE_Phoenix_MotorControl_Set.vi"("Output"=w352, "Control Mode"=w351, "PhoenixMotorControlDevRef"=w353) -> ()  [unwired: 7 in, 2 out]
                n149 = call "CTRE_Phoenix_MotorControl_Set.vi"("Output"=w352, "Control Mode"=w351, "PhoenixMotorControlDevRef"=w356) -> ()  [unwired: 7 in, 2 out]
                n150 = call "CTRE_Phoenix_MotorControl_Set.vi"("Output"=w352, "Control Mode"=w351, "PhoenixMotorControlDevRef"=w355) -> ()  [unwired: 7 in, 2 out]
              }
            }
          }
          frame condition #2 {
          }
        }
        n151 = Less Or Equal To 0?(x=w308) -> (x <= 0?=w299:bool)
        n152 = Max & Min(x=w308, y=25.0) -> (min(x,y)=w304:dbl)  [unwired: 1 out]
        n153 = Or(x=w298, y=w299) -> (x .or. y?=w300:bool)
      }
      frame "Puke" {
        # "How much longer?\nUpdate motors every 25ms till time runs out OR\nsensor trips"
        n154 = Unbundle(w374) -> ("Start Time (ms)"=w377:u32, "Iterations"=w361:i32)
        n155 = Equal?(x=w361, y=0 ("value")) -> (x = y?=w359:bool)
        n156 = Subtract(x=w373, y=w377) -> (x-y=w380:u32)
        n157 = Multiply(x=w369, y=1000.0) -> (x*y=w379:dbl)
        n158 = case shown="True" w359 {
          tunnel: w358 -> [w381 w384]
          tunnel: [w381 w382] -> w357
          frame False {
          }
          frame True {
            n159 = call <vilib>:"WPI_AnalogTriggerGetOutput.vi"("AnalogTriggerDevRef"=w384) -> ("Trigger State"=→"WaitTrigger":bool, "AnalogTriggerDevRef"=w382:T11)  [unwired: 7 in, 2 out]
          }
        }
        n160 = disable-structure shown="robot_simulation==off" {
          disable-tunnel: w371 -> [w392 w419 _]
          disable-tunnel: w370 -> [w387 w414 _]
          disable-tunnel: w365 -> [w391 w418 _]
          disable-tunnel: w362 -> [_ _ _]
          disable-tunnel: [w390 w417 _] -> w366
          disable-tunnel: w364 -> [w393 w420 _]
          disable-tunnel: w363 -> [w389 w416 _]
          disable-tunnel: w357 -> [w386 w413 _]
          frame condition #0 (active) {
            n161 = local read "WaitTrigger"() -> (w388:bool)
            n162 = case shown="True" w388 {
              tunnel: w386 -> [w395 w398]
              tunnel: [w394 FALSE ("Trigger State")] -> w385
              frame False {
                n163 = call <vilib>:"WPI_AnalogTriggerGetOutput.vi"("AnalogTriggerDevRef"=w395) -> ("Trigger State"=w394:bool)  [unwired: 7 in, 3 out]
              }
              frame True {
                n164 = call <vilib>:"WPI_AnalogTriggerGetOutput.vi"("AnalogTriggerDevRef"=w398) -> ("Trigger State"=w396:bool)  [unwired: 7 in, 3 out]
                n165 = local write "WaitTrigger"(w396) -> ()
              }
            }
            n166 = case shown="False" w385 {
              tunnel: w392 -> [w404 w410]
              tunnel: w387 -> [w403 w409]
              tunnel: w391 -> [_ w406]
              tunnel: [TRUE FALSE] -> w390
              tunnel: w393 -> [w401 w408]
              tunnel: w389 -> [_ w405]
              frame True {
                w399 = T16 0 items=["PercentOutput"=0, "Position"=1, "Velocity"=2, "Current"=3, "Follower"=5, "MotionProfile"=6, "MotionMagic"=7, "MotionMagicArc"=8, "MotionProfileArc"=10, "Disabled"=15] ("Control Mode")
                w400 = 0.0 ("Output")
                n167 = call "CTRE_Phoenix_MotorControl_Set.vi"("Output"=w400, "Control Mode"=w399, "PhoenixMotorControlDevRef"=w401) -> ()  [unwired: 7 in, 2 out]
                n168 = call "CTRE_Phoenix_MotorControl_Set.vi"("Output"=w400, "Control Mode"=w399, "PhoenixMotorControlDevRef"=w404) -> ()  [unwired: 7 in, 2 out]
                n169 = call "CTRE_Phoenix_MotorControl_Set.vi"("Output"=w400, "Control Mode"=w399, "PhoenixMotorControlDevRef"=w403) -> ()  [unwired: 7 in, 2 out]
              }
              frame False {
                w407 = T16 0 items=["PercentOutput"=0, "Position"=1, "Velocity"=2, "Current"=3, "Follower"=5, "MotionProfile"=6, "MotionMagic"=7, "MotionMagicArc"=8, "MotionProfileArc"=10, "Disabled"=15] ("Control Mode")
                n170 = call "CTRE_Phoenix_MotorControl_Set.vi"("Output"=w406, "Control Mode"=w407, "PhoenixMotorControlDevRef"=w410) -> ()  [unwired: 7 in, 2 out]
                n171 = call "CTRE_Phoenix_MotorControl_Set.vi"("Output"=w406, "Control Mode"=w407, "PhoenixMotorControlDevRef"=w409) -> ()  [unwired: 7 in, 2 out]
                n172 = call "CTRE_Phoenix_MotorControl_Set.vi"("Output"=w405, "Control Mode"=w407, "PhoenixMotorControlDevRef"=w408) -> ()  [unwired: 7 in, 2 out]
              }
            }
          }
          frame condition #1 {
            n173 = local read "WaitTrigger"() -> (w415:bool)
            n174 = case shown="True" w415 {
              tunnel: w413 -> [w422 w425]
              tunnel: [w421 FALSE ("Trigger State")] -> w412
              frame False {
                n175 = call <vilib>:"WPI_AnalogTriggerGetOutput.vi"("AnalogTriggerDevRef"=w422) -> ("Trigger State"=w421:bool)  [unwired: 7 in, 3 out]
              }
              frame True {
                n176 = call <vilib>:"WPI_AnalogTriggerGetOutput.vi"("AnalogTriggerDevRef"=w425) -> ("Trigger State"=w423:bool)  [unwired: 7 in, 3 out]
                n177 = local write "WaitTrigger"(w423) -> ()
              }
            }
            n178 = case shown="False" w412 {
              tunnel: w419 -> [w431 w439]
              tunnel: w414 -> [w430 w438]
              tunnel: w418 -> [_ w433]
              tunnel: [TRUE FALSE] -> w417
              tunnel: w420 -> [w428 w437]
              tunnel: w416 -> [_ w435]
              frame True {
                w426 = T16 0 items=["PercentOutput"=0, "Position"=1, "Velocity"=2, "Current"=3, "Follower"=5, "MotionProfile"=6, "MotionMagic"=7, "MotionMagicArc"=8, "MotionProfileArc"=10, "Disabled"=15] ("Control Mode")
                w427 = 0.0 ("Output")
                n179 = call "CTRE_Phoenix_MotorControl_Set.vi"("Output"=w427, "Control Mode"=w426, "PhoenixMotorControlDevRef"=w428) -> ()  [unwired: 7 in, 2 out]
                n180 = call "CTRE_Phoenix_MotorControl_Set.vi"("Output"=w427, "Control Mode"=w426, "PhoenixMotorControlDevRef"=w431) -> ()  [unwired: 7 in, 2 out]
                n181 = call "CTRE_Phoenix_MotorControl_Set.vi"("Output"=w427, "Control Mode"=w426, "PhoenixMotorControlDevRef"=w430) -> ()  [unwired: 7 in, 2 out]
              }
              frame False {
                w436 = T16 0 items=["PercentOutput"=0, "Position"=1, "Velocity"=2, "Current"=3, "Follower"=5, "MotionProfile"=6, "MotionMagic"=7, "MotionMagicArc"=8, "MotionProfileArc"=10, "Disabled"=15] ("Control Mode")
                n182 = Negate(x=w435) -> (-x=w434:dbl)
                n183 = Negate(x=w433) -> (-x=w432:dbl)
                n184 = call "CTRE_Phoenix_MotorControl_Set.vi"("Output"=w432, "Control Mode"=w436, "PhoenixMotorControlDevRef"=w439) -> ()  [unwired: 7 in, 2 out]
                n185 = call "CTRE_Phoenix_MotorControl_Set.vi"("Output"=w432, "Control Mode"=w436, "PhoenixMotorControlDevRef"=w438) -> ()  [unwired: 7 in, 2 out]
                n186 = call "CTRE_Phoenix_MotorControl_Set.vi"("Output"=w434, "Control Mode"=w436, "PhoenixMotorControlDevRef"=w437) -> ()  [unwired: 7 in, 2 out]
              }
            }
          }
          frame condition #2 {
          }
        }
        n187 = Subtract(x=w379, y=w380) -> (x-y=w376:dbl)
        n188 = Less Or Equal To 0?(x=w376) -> (x <= 0?=w367:bool)
        n189 = Max & Min(x=w376, y=25.0) -> (min(x,y)=w372:dbl)  [unwired: 1 out]
        n190 = Or(x=w366, y=w367) -> (x .or. y?=w368:bool)
      }
    }
    n191 = call "cube Check for New Command.vi"("Current Command"=w76, "Wait time (ms)"=w81, "Finished?"=w82) -> ("Completion"=w77:T1, "Subsystem Name"=w78:string, "Current Command"=w79:T2, "Initial Trace String"=w80:string, "NextCommand"=w83:T15)  [unwired: 4 in]
    n192 = case shown="\"Successful\", \"Aborted\"" w77 {
      selector: w77 -> [_ w104]
      tunnel: w80 -> [_ w100]
      tunnel: w79 -> [_ w101]
      tunnel: w78 -> [_ w98]
      frame "Incomplete", Default {
        # "Continuing current command"
      }
      frame "Successful", "Aborted" {
        # "Report and setup for next command"
        n193 = Unbundle By Name(w101) -> ("Arm Setpoint"=w103:dbl, "Duration"=w97:dbl, "Conveyor Setpoint"=w96:dbl)
        n194 = Format Into String(format string="A %.1f, C %.1f, D %f", initial string=w100, w103, w96, w97) -> (resulting string=w99:string)  [unwired: 1 in, 1 out]
        "Current\nCmd" <- w99
        n195 = call <vilib>:"Trace Results.vi"("Status of previous command"=w104, "Description"=w99, "Subsystem"=w98) -> ()  [unwired: 9 in]
      }
    }
    n196 = disable-structure shown="Disabled" {
      frame Disabled {
        # "Publish"
        n197 = call-poly <vilib>:"NT Write Value.vi"() -> ()  [unwired: 11 in, 1 out]
      }
      frame Enabled {
      }
    }
  }
